vi "FFT.vi"(3 "Y":dbl[](array[numeric]), 5 "dt":dbl) -> (0 "FFT Señal":cluster{dbl, dbl, dbl[]}(graph), 1 "FFT {X}":cdb[](array[numeric]), 2 "df":dbl)   [LabVIEW 2021]
uses:
  <vilib>/Analysis/NI_AALPro.lvlib
panel:
  out "Substraccion . Real de F(X)/Tamaño de la señal 2":dbl[](graph)
  out "Tamaño/2.0 a I32":i32
  out "Real de F(X)/Tamaño de la señal":dbl[](graph)
  out "Tamaño*dt":dbl
  out "Tamaño/2.0":dbl
  out "F(X)":dbl[](graph)
  out "Tamaño de la señal":i32
  out "Real de F(X)":dbl[](graph)
  # "df=1/Tamaño*dt"
  # "Obtengo los valores de la señal y su grafica."
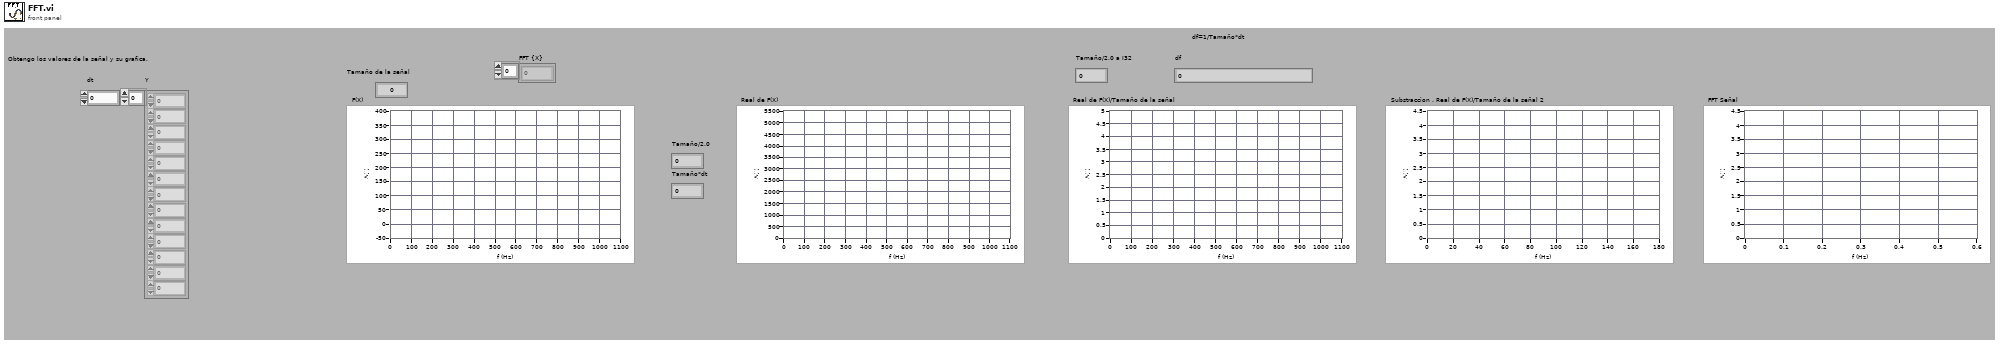
[diagram p1: front panel]
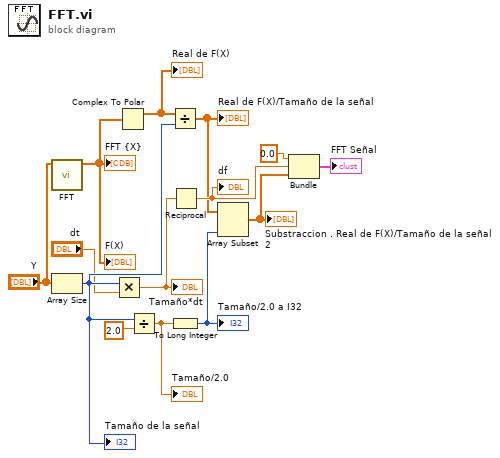
[diagram p0: block diagram]
diagram:
  n1 = call-poly <vilib>:"FFT.vi"("X"="Y") -> ("FFT {X}"=w5:cdb[])  [unwired: 9 in, 1 out]
  "F(X)" <- w5
  "FFT {X}" <- w5
  n2 = Array Size(array="Y") -> (size(s)=w10:i32)
  "Tamaño de la señal" <- w10
  n3 = Multiply(x=w10, y="dt") -> (x*y=w9:dbl)
  "Tamaño*dt" <- w9
  n4 = Complex To Polar(r * e^(i*theta)=w5) -> (r=w14:dbl[])  [unwired: 1 out]
  "Real de F(X)" <- w14
  n5 = Divide(x=w10, y=2.0) -> (x/y=w7:dbl)
  "Tamaño/2.0" <- w7
  n6 = Divide(x=w14, y=w10) -> (x/y=w4:dbl[])
  "Real de F(X)/Tamaño de la señal" <- w4
  n7 = To Long Integer(number=w7) -> (32bit integer=w8:i32)
  "Tamaño/2.0 a I32" <- w8
  n8 = Reciprocal(x=w9) -> (1/x=w12:dbl)
  "df" <- w12
  n9 = Array Subset(array=w4, length=w8) -> (w3:dbl[])  [unwired: 1 in]
  "Substraccion . Real de F(X)/Tamaño de la señal 2" <- w3
  n10 = Bundle(0.0, w12, w3) -> (→"FFT Señal":cluster{dbl, dbl, dbl[]})  [unwired: 1 in]
